vi "Grade IO Test.vi"(8 "Data Map":T5(array[cluster]) {"OPC UA Data Type" items=["Boolean"=1, "SByte"=2, "Byte"=3, "Int16"=4, "UInt16"=5, "Int32"=6, "UInt32"=7, "Int64"=8, "UInt64"=9, "Float"=10, "Double"=11, "String"=12, "DateTime"=13, "ByteString"=15, "Array of Boolean"=101, "Array of SByte"=102, "Array of Byte"=103, "Array of Int16"=104, "Array of UInt16"=105, "Array of Int32"=106, "Array of UInt32"=107, "Array of Int64"=108, "Array of UInt64"=109, "Array of Float"=110, "Array of Double"=111, "Array of String"=112, "Array of DateTime"=113, "Array of ByteString"=115]}, 9 "Server Data":T1(array[cluster]), 10 "data table in":T2) -> (2 "Pass?":bool[](array[boolean]))   [LabVIEW 2013, in "OPC UA Client Tests.lvlib"]
doc: "Checks to see that the Server Data (data written using OPC UA Server API) matches what is in the module's data table. Input map is used to map data table items to server data items."
uses:
  OPC UA Client Tests.lvlib
  <vilib>/NI/Tag Bus/tag/Data Type.ctl
  module/configuration/OPC UA Data Type.ctl
  <vilib>/NI/Tag Bus/table/data table.ctl
  <vilib>/NI/Tag Bus/table/data polymorphs/read one/read Boolean.vi
  <vilib>/NI/Tag Bus/table/data polymorphs/read one/read I8.vi
  <vilib>/NI/Tag Bus/table/data polymorphs/read one/read U8.vi
  <vilib>/NI/Tag Bus/table/data polymorphs/read one/read I16.vi
  <vilib>/NI/Tag Bus/table/data polymorphs/read one/read U16.vi
  <vilib>/NI/Tag Bus/table/data polymorphs/read one/read I32.vi
  <vilib>/NI/Tag Bus/table/data polymorphs/read one/read U32.vi
  <vilib>/NI/Tag Bus/table/data polymorphs/read one/read I64.vi
  <vilib>/NI/Tag Bus/table/data polymorphs/read one/read U64.vi
  <vilib>/NI/Tag Bus/table/data polymorphs/read one/read Single.vi
  <vilib>/NI/Tag Bus/table/data polymorphs/read one/read Double.vi
  <vilib>/NI/Tag Bus/table/data polymorphs/read one/read String.vi
  <vilib>/NI/Tag Bus/table/data polymorphs/read one/read Array of Boolean.vi
  <vilib>/NI/Tag Bus/table/data polymorphs/read one/read Array of I8.vi
  <vilib>/NI/Tag Bus/table/data polymorphs/read one/read Array of U8.vi
  <vilib>/NI/Tag Bus/table/data polymorphs/read one/read Array of I16.vi
  <vilib>/NI/Tag Bus/table/data polymorphs/read one/read Array of U16.vi
  <vilib>/NI/Tag Bus/table/data polymorphs/read one/read Array of I32.vi
  <vilib>/NI/Tag Bus/table/data polymorphs/read one/read Array of U32.vi
  <vilib>/NI/Tag Bus/table/data polymorphs/read one/read Array of I64.vi
  <vilib>/NI/Tag Bus/table/data polymorphs/read one/read Array of U64.vi
  <vilib>/NI/Tag Bus/table/data polymorphs/read one/read Array of Single.vi
  <vilib>/NI/Tag Bus/table/data polymorphs/read one/read Array of Double.vi
  <vilib>/NI/Tag Bus/table/data polymorphs/read one/read Array of String.vi
  <vilib>/NI/Tag Bus/table/data table.lvlib
  module/execution/OPC UA Client runtime.lvclass
  <vilib>/NI/Tag Bus/tag/tag descriptor.lvclass
  module/configuration/OPC UA Client configuration.lvclass
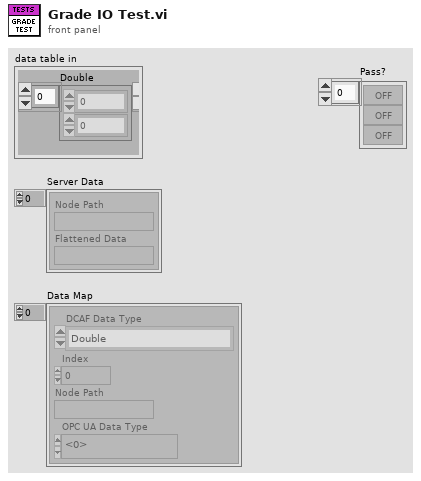
[diagram p1: front panel]
types:
  T1 = cluster{"Node Path":string, "Flattened Data":string}[]
  T2 = typedef "tag bus.lvlib/data table.lvlib/data table.ctl" = cluster{"Double":dbl[], "Single":sgl[], "I64":i64[], "I32":i32[], "I16":i16[], "I8":i8[], "U64":u64[], "U32":u32[], "U16":u16[], "U8":u8[], "Boolean":bool[], "String":string[], "Array of Double":cluster{"DBL Array":dbl[]}[], "Array of Single":cluster{"SGL Array":sgl[]}[], "Array of I64":cluster{"I64 Array":i64[]}[], "Array of I32":cluster{"I32 Array":i32[]}[], "Array of I16":cluster{"I16 Array":i16[]}[], "Array of I8":cluster{"I8 Array":i8[]}[], "Array of U64":cluster{"U64 Array":u64[]}[], "Array of U32":cluster{"U32 Array":u32[]}[], "Array of U16":cluster{"U16 Array":u16[]}[], "Array of U8":cluster{"U8 Array":u8[]}[], "Array of Boolean":cluster{"Boolean Array":bool[]}[], "Array of String":cluster{"String Array":string[]}[]}
  T3 = typedef "tag bus.lvlib/tag descriptor.lvclass/Data Type.ctl" = enum16{"Double", "Single", "I64", "I32", "I16", "I8", "U64", "U32", "U16", "U8", "Boolean", "String", "Array of Double", "Array of Single", "Array of I64", "Array of I32", "Array of I16", "Array of I8", "Array of U64", "Array of U32", "Array of U16", "Array of U8", "Array of Boolean", "Array of String"}
  T4 = typedef "OPC UA Client configuration.lvclass/OPC UA Data Type.ctl" = u16
  T5 = cluster{"DCAF Data Type":T3, "Index":i32, "Node Path":string, "OPC UA Data Type":T4}[]
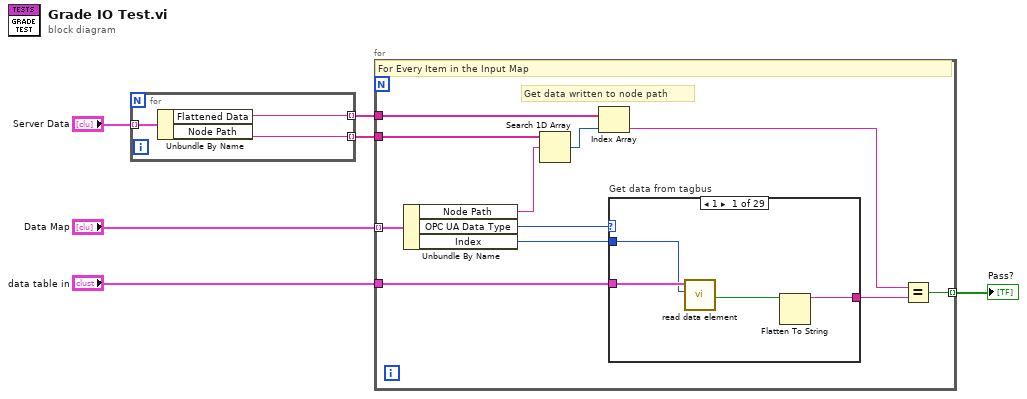
[diagram p0: block diagram]
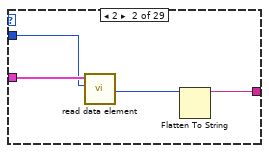
[diagram p2: hidden frame]
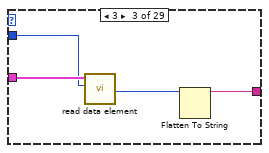
[diagram p3: hidden frame]
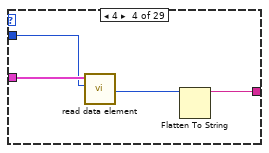
[diagram p4: hidden frame]
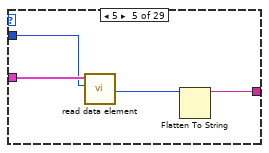
[diagram p5: hidden frame]
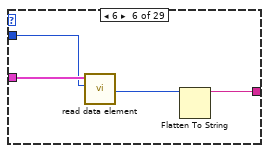
[diagram p6: hidden frame]
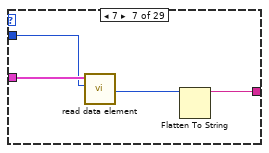
[diagram p7: hidden frame]
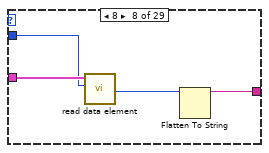
[diagram p8: hidden frame]
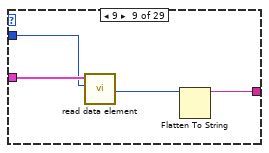
[diagram p9: hidden frame]
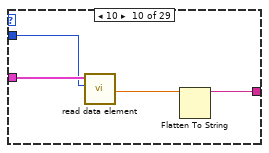
[diagram p10: hidden frame]
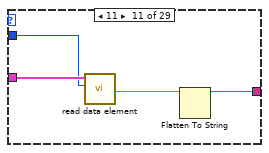
[diagram p11: hidden frame]
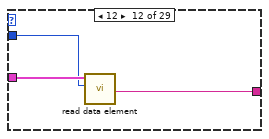
[diagram p12: hidden frame]
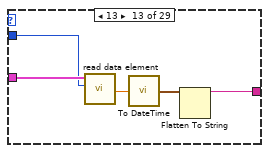
[diagram p13: hidden frame]
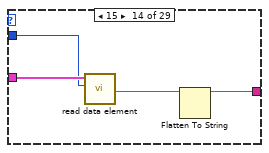
[diagram p14: hidden frame]
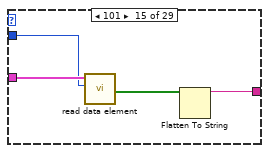
[diagram p15: hidden frame]
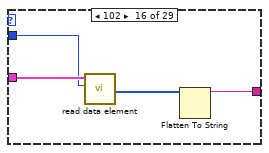
[diagram p16: hidden frame]
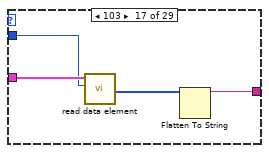
[diagram p17: hidden frame]
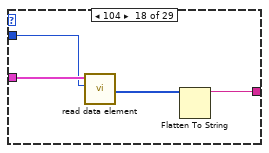
[diagram p18: hidden frame]
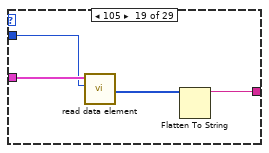
[diagram p19: hidden frame]
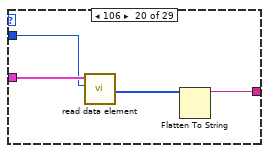
[diagram p20: hidden frame]
diagram:
  n1 = for {
    tunnel: "Server Data" -> [w9] mode=indexing
    tunnel: [w8] -> w3 mode=indexing
    tunnel: [w7] -> w2 mode=indexing
    n2 = Unbundle By Name(w9) -> ("Flattened Data"=w8:string, "Node Path"=w7:string)
  }
  n3 = for {
    tunnel: "Data Map" -> [w20] mode=indexing
    tunnel: "data table in" -> [w18]
    tunnel: w3 -> [w13]
    tunnel: w2 -> [w15]
    tunnel: [w10] -> w1 mode=indexing
    # "Get data written to node path"
    # "For Every Item in the Input Map"
    n4 = Unbundle By Name(w20) -> ("Node Path"=w16:string, "OPC UA Data Type"=w17:T4, "Index"=w19:i32)
    n5 = Search 1D Array(1D array=w15, element=w16) -> (index of element=w14:i32)  [unwired: 1 in]
    n6 = Index Array(array=w13, index=w14) -> (element=w11:string)
    n7 = case "Get data from tagbus" shown="1" w17 {
      tunnel: w19 -> [w23 w27 w31 w35 w39 w43 w47 w51 w55 w59 w63 w66 w71 w75 w79 w83 w87 w91 w95 w99 w103 w107 w111 w115 w119 w123 w128 w132 _]
      tunnel: w18 -> [w24 w28 w32 w36 w40 w44 w48 w52 w56 w60 w64 w67 w72 w76 w80 w84 w88 w92 w96 w100 w104 w108 w112 w116 w120 w124 w129 w133 _]
      tunnel: [w21 w25 w29 w33 w37 w41 w45 w49 w53 w57 w61 w65 w70 w73 w77 w81 w85 w89 w93 w97 w101 w105 w109 w113 w117 w121 w127 w130 "" ("data string")] -> w12
      frame 1 {
        n8 = call-poly <vilib>:"read data element.vi"("index"=w23, "data table in"=w24) -> ("value"=w22:bool)  [unwired: 8 in, 1 out]
        n9 = Flatten To String(anything=w22) -> (data string=w21:string)  [unwired: 3 in, 2 out]
      }
      frame 2 {
        n10 = call-poly <vilib>:"read data element.vi"("index"=w27, "data table in"=w28) -> ("value"=w26:i8)  [unwired: 8 in, 1 out]
        n11 = Flatten To String(anything=w26) -> (data string=w25:string)  [unwired: 3 in, 2 out]
      }
      frame 3 {
        n12 = call-poly <vilib>:"read data element.vi"("index"=w31, "data table in"=w32) -> ("value"=w30:u8)  [unwired: 8 in, 1 out]
        n13 = Flatten To String(anything=w30) -> (data string=w29:string)  [unwired: 3 in, 2 out]
      }
      frame 4 {
        n14 = call-poly <vilib>:"read data element.vi"("index"=w35, "data table in"=w36) -> ("value"=w34:i16)  [unwired: 8 in, 1 out]
        n15 = Flatten To String(anything=w34) -> (data string=w33:string)  [unwired: 3 in, 2 out]
      }
      frame 5 {
        n16 = call-poly <vilib>:"read data element.vi"("index"=w39, "data table in"=w40) -> ("value"=w38:u16)  [unwired: 8 in, 1 out]
        n17 = Flatten To String(anything=w38) -> (data string=w37:string)  [unwired: 3 in, 2 out]
      }
      frame 6 {
        n18 = call-poly <vilib>:"read data element.vi"("index"=w43, "data table in"=w44) -> ("value"=w42:i32)  [unwired: 8 in, 1 out]
        n19 = Flatten To String(anything=w42) -> (data string=w41:string)  [unwired: 3 in, 2 out]
      }
      frame 7 {
        n20 = call-poly <vilib>:"read data element.vi"("index"=w47, "data table in"=w48) -> ("value"=w46:u32)  [unwired: 8 in, 1 out]
        n21 = Flatten To String(anything=w46) -> (data string=w45:string)  [unwired: 3 in, 2 out]
      }
      frame 8 {
        n22 = call-poly <vilib>:"read data element.vi"("index"=w51, "data table in"=w52) -> ("value"=w50:i64)  [unwired: 8 in, 1 out]
        n23 = Flatten To String(anything=w50) -> (data string=w49:string)  [unwired: 3 in, 2 out]
      }
      frame 9 {
        n24 = call-poly <vilib>:"read data element.vi"("index"=w55, "data table in"=w56) -> ("value"=w54:u64)  [unwired: 8 in, 1 out]
        n25 = Flatten To String(anything=w54) -> (data string=w53:string)  [unwired: 3 in, 2 out]
      }
      frame 10 {
        n26 = call-poly <vilib>:"read data element.vi"("index"=w59, "data table in"=w60) -> ("value"=w58:sgl)  [unwired: 8 in, 1 out]
        n27 = Flatten To String(anything=w58) -> (data string=w57:string)  [unwired: 3 in, 2 out]
      }
      frame 11 {
        n28 = call-poly <vilib>:"read data element.vi"("index"=w63, "data table in"=w64) -> ("value"=w62:dbl)  [unwired: 8 in, 1 out]
        n29 = Flatten To String(anything=w62) -> (data string=w61:string)  [unwired: 3 in, 2 out]
      }
      frame 12 {
        n30 = call-poly <vilib>:"read data element.vi"("index"=w66, "data table in"=w67) -> ("value"=w65:string)  [unwired: 8 in, 1 out]
      }
      frame 13 {
        n31 = call-poly <vilib>:"read data element.vi"("index"=w71, "data table in"=w72) -> ("value"=w68:dbl)  [unwired: 8 in, 1 out]
        n32 = call "To DateTime.vi"("Formatted DateTime"=w68) -> ("Time Stamp"=w69:timestamp)
        n33 = Flatten To String(anything=w69) -> (data string=w70:string)  [unwired: 3 in, 2 out]
      }
      frame 15 {
        n34 = call-poly <vilib>:"read data element.vi"("index"=w75, "data table in"=w76) -> ("value"=w74:string)  [unwired: 8 in, 1 out]
        n35 = Flatten To String(anything=w74) -> (data string=w73:string)  [unwired: 3 in, 2 out]
      }
      frame 101 {
        n36 = call-poly <vilib>:"read data element.vi"("index"=w79, "data table in"=w80) -> ("value"=w78:bool[])  [unwired: 8 in, 1 out]
        n37 = Flatten To String(anything=w78) -> (data string=w77:string)  [unwired: 3 in, 2 out]
      }
      frame 102 {
        n38 = call-poly <vilib>:"read data element.vi"("index"=w83, "data table in"=w84) -> ("value"=w82:i8[])  [unwired: 8 in, 1 out]
        n39 = Flatten To String(anything=w82) -> (data string=w81:string)  [unwired: 3 in, 2 out]
      }
      frame 103 {
        n40 = call-poly <vilib>:"read data element.vi"("index"=w87, "data table in"=w88) -> ("value"=w86:u8[])  [unwired: 8 in, 1 out]
        n41 = Flatten To String(anything=w86) -> (data string=w85:string)  [unwired: 3 in, 2 out]
      }
      frame 104 {
        n42 = call-poly <vilib>:"read data element.vi"("index"=w91, "data table in"=w92) -> ("value"=w90:i16[])  [unwired: 8 in, 1 out]
        n43 = Flatten To String(anything=w90) -> (data string=w89:string)  [unwired: 3 in, 2 out]
      }
      frame 105 {
        n44 = call-poly <vilib>:"read data element.vi"("index"=w95, "data table in"=w96) -> ("value"=w94:u16[])  [unwired: 8 in, 1 out]
        n45 = Flatten To String(anything=w94) -> (data string=w93:string)  [unwired: 3 in, 2 out]
      }
      frame 106 {
        n46 = call-poly <vilib>:"read data element.vi"("index"=w99, "data table in"=w100) -> ("value"=w98:i32[])  [unwired: 8 in, 1 out]
        n47 = Flatten To String(anything=w98) -> (data string=w97:string)  [unwired: 3 in, 2 out]
      }
      frame 107 {
        n48 = call-poly <vilib>:"read data element.vi"("index"=w103, "data table in"=w104) -> ("value"=w102:u32[])  [unwired: 8 in, 1 out]
        n49 = Flatten To String(anything=w102) -> (data string=w101:string)  [unwired: 3 in, 2 out]
      }
      frame 108 {
        n50 = call-poly <vilib>:"read data element.vi"("index"=w107, "data table in"=w108) -> ("value"=w106:i64[])  [unwired: 8 in, 1 out]
        n51 = Flatten To String(anything=w106) -> (data string=w105:string)  [unwired: 3 in, 2 out]
      }
      frame 109 {
        n52 = call-poly <vilib>:"read data element.vi"("index"=w111, "data table in"=w112) -> ("value"=w110:u64[])  [unwired: 8 in, 1 out]
        n53 = Flatten To String(anything=w110) -> (data string=w109:string)  [unwired: 3 in, 2 out]
      }
      frame 110 {
        n54 = call-poly <vilib>:"read data element.vi"("index"=w115, "data table in"=w116) -> ("value"=w114:sgl[])  [unwired: 8 in, 1 out]
        n55 = Flatten To String(anything=w114) -> (data string=w113:string)  [unwired: 3 in, 2 out]
      }
      frame 111 {
        n56 = call-poly <vilib>:"read data element.vi"("index"=w119, "data table in"=w120) -> ("value"=w118:dbl[])  [unwired: 8 in, 1 out]
        n57 = Flatten To String(anything=w118) -> (data string=w117:string)  [unwired: 3 in, 2 out]
      }
      frame 112 {
        n58 = call-poly <vilib>:"read data element.vi"("index"=w123, "data table in"=w124) -> ("value"=w122:string[])  [unwired: 8 in, 1 out]
        n59 = Flatten To String(anything=w122) -> (data string=w121:string)  [unwired: 3 in, 2 out]
      }
      frame 113 {
        n60 = call-poly <vilib>:"read data element.vi"("index"=w128, "data table in"=w129) -> ("value"=w126:dbl[])  [unwired: 8 in, 1 out]
        n61 = call "To DateTime Array.vi"("Formatted DateTime Array"=w126) -> ("DateTime Array"=w125:timestamp[])
        n62 = Flatten To String(anything=w125) -> (data string=w127:string)  [unwired: 3 in, 2 out]
      }
      frame 115 {
        n63 = call-poly <vilib>:"read data element.vi"("index"=w132, "data table in"=w133) -> ("value"=w131:string[])  [unwired: 8 in, 1 out]
        n64 = Flatten To String(anything=w131) -> (data string=w130:string)  [unwired: 3 in, 2 out]
      }
      frame 0, Default {
      }
    }
    n65 = Equal?(x=w11, y=w12) -> (x = y?=w10:bool)
  }
  "Pass?" <- w1
